vi "Configure X Axis For Segment Sweep.vi"(7 "Channel (1)":i32=1, 8 "error in (no error)":errorcluster, 10 "Display Method (0: Linear)":i32(ring) items=["Linear", "Order Base"], 11 "VISA resource name":refnum<visa-resource-name>) -> (0 "error out":errorcluster, 3 "VISA resource name out":refnum<visa-resource-name>)   [LabVIEW 2018, in "Agilent ENA Series.lvlib"]
doc: "Selects the display method of the graph horizontal axis of selected channel for segment sweep."
uses:
  Agilent ENA Series.lvlib
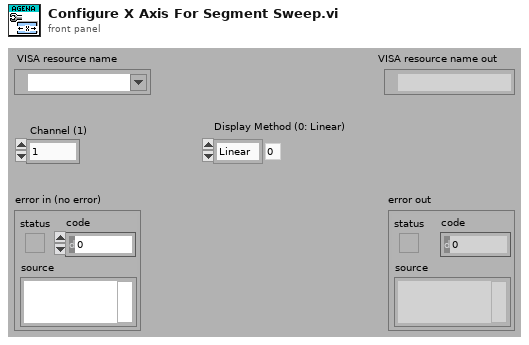
[diagram p1: front panel]
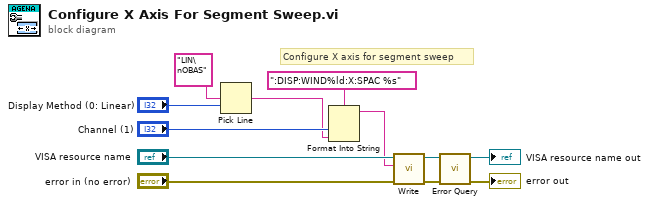
[diagram p0: block diagram]
diagram:
  # "Configure X axis for segment sweep"
  n1 = Pick Line(multi-line string="LIN\nOBAS", line index="Display Method (0: Linear)") -> (output string=w6:string)  [unwired: 1 in]
  n2 = Format Into String(format string=":DISP:WIND%ld:X:SPAC %s", "Channel (1)", w6) -> (resulting string=w5:string)  [unwired: 2 in, 1 out]
  n3 = call "Write.vi"("error in (no error)"="error in (no error)", "String ()"=w5, "VISA resource name"="VISA resource name") -> ("error out"=w3:errorcluster, "VISA resource name out"=w4:refnum<visa-resource-name>)  [unwired: 6 in, 1 out]
  n4 = call "Error Query.vi"("error in (no error)"=w3, "VISA resource name"=w4) -> ("error out"=→"error out":errorcluster, "VISA resource name out"=→"VISA resource name out":refnum<visa-resource-name>)  [unwired: 6 in, 2 out]
